vi "Build Delete Parameters.vi"(4 "TypeMap in":refnum<class "TypeMap.lvclass">, 8 "error in (no error)":errorcluster, 10 "object":variant, 11 "SqlMapper in":refnum<class "SqlMapper.lvclass">) -> (0 "error out":errorcluster, 1 "DynamicParameters out":refnum<class "DynamicParameters.lvclass">, 3 "SqlMapper out":refnum<class "SqlMapper.lvclass">)   [LabVIEW 2020, in "ORM.lvlib" / "TypeMap.lvclass"]
uses:
  TypeMap.lvclass
  DynamicParameters/DynamicParameters.lvclass
  SqlMapper/SqlMapper.lvclass
  TypeMap.lvclass/TypeMap.ctl
  DynamicParameters/DynamicParameters.lvclass/DynamicParameters.ctl
  DynamicParameters/Write KeyProperties.vi
  Read Autokey.vi
  Read KeyProperties.vi
  <vilib>/Utility/error.llb/Error Cluster From Error Code.vi
  <vilib>/ErrorRing/Error Ring.xnode
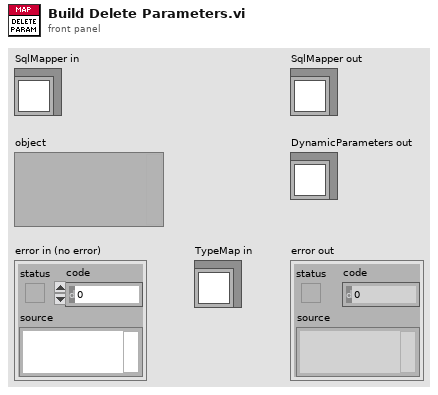
[diagram p1: front panel]
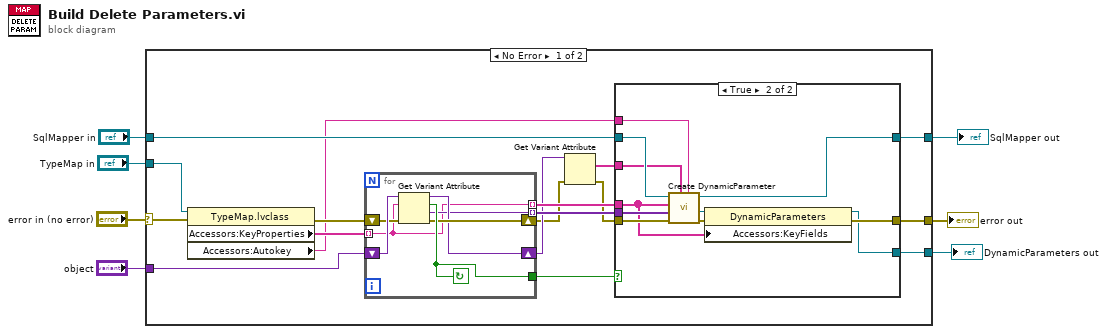
[diagram p0: block diagram]
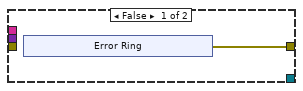
[diagram p2: hidden frame]
diagram:
  n1 = case shown="No Error" "error in (no error)" {
    selector: "error in (no error)" -> [w22 w49]
    tunnel: "TypeMap in" -> [w21 _]
    tunnel: "object" -> [w13 _]
    tunnel: "SqlMapper in" -> [w18 w50]
    tunnel: [w16 w50] -> w3
    tunnel: [w15 w49] -> w2
    tunnel: [w14 _] -> w1
    frame No Error {
      n2 = property class="TypeMap.lvclass"(reference=w21, error in=w22) -> (error out=w23:errorcluster, "Accessors:KeyProperties"=w24:string[], "Accessors:Autokey"=w11:string)  [unwired: 1 out]
      n3 = for {
        tunnel: w24 -> [w25] mode=indexing
        tunnel: [w30] -> w17
        shift-right: [w29] -> w9
        shift-left: w23 -> [w28]
        shift-right: [w27] -> w10
        shift-left: w13 -> [w31]
        tunnel: [w26] -> w20 mode=indexing
        tunnel: [w25] -> w19 mode=indexing
        stop <- w30 continue-if-true
        n4 = Get Variant Attribute(Variant=w31, name=w25, error in=w28) -> (duplicate Variant=w27:variant, found=w30:bool, value=w26:variant, error out=w29:errorcluster)  [unwired: 1 in]
      }
      n5 = Get Variant Attribute(Variant=w10, error in=w9) -> (names=w12:string[], error out=w8:errorcluster)  [unwired: 2 in, 2 out]
      n6 = case shown="True" w17 {
        tunnel: w8 -> [_ w48]
        tunnel: w20 -> [_ w47]
        tunnel: w19 -> [_ w38]
        tunnel: w18 -> [_ w46]
        tunnel: [_ w45] -> w16
        tunnel: [w32 w41] -> w15
        tunnel: [_ w39] -> w14
        tunnel: w12 -> [_ w43]
        tunnel: w11 -> [_ w42]
        frame False {
          n7 = xnode "Error Ring"() -> ("error out"=w32:errorcluster)
        }
        frame True {
          n8 = call "Create DynamicParameter.vi"("AutoKey"=w42, "RequestedFields"=w43, "error in (no error)"=w48, "ParameterValues"=w47, "ParameterNames"=w38, "SqlMapper in"=w46) -> ("error out"=w44:errorcluster, "Parameters"=w40:refnum<class "DynamicParameters.lvclass">, "SqlMapper out"=w45:refnum<class "SqlMapper.lvclass">)  [unwired: 1 in, 2 out]
          n9 = property class="DynamicParameters"(reference=w40, error in=w44, "Accessors:KeyFields"=w38) -> (reference out=w39:refnum<class "DynamicParameters.lvclass">, error out=w41:errorcluster)
        }
      }
    }
    frame Error {
    }
  }
  "error out" <- w2
  "SqlMapper out" <- w3
  "DynamicParameters out" <- w1
